vi "Prepare_Error_Array(SubVI).vi"(9 "Value":dbl, 10 "Info":dbl, 11 "Array in":string[](array[string])) -> (3 "Array out":string[](array[string]))   [LabVIEW 2017]
doc: "SubVI that update string array containing error list that i displayed on main window."
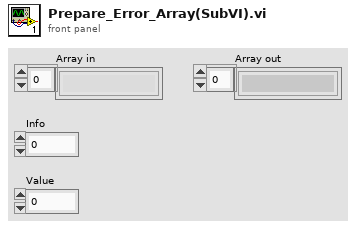
[diagram p1: front panel]
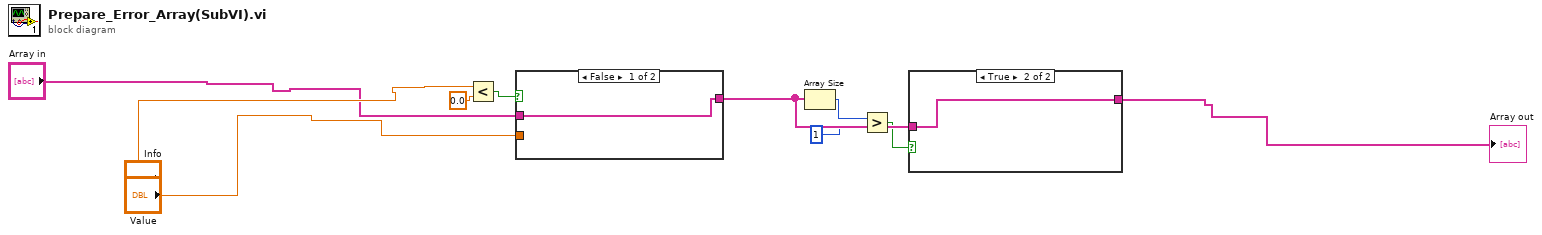
[diagram p0: block diagram]
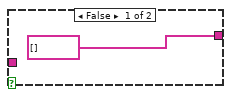
[diagram p2: hidden frame]
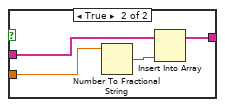
[diagram p3: hidden frame]
diagram:
  n1 = Less?(x="Info", y=0.0) -> (x < y?=w5:bool)
  n2 = case shown="False" w5 {
    tunnel: "Array in" -> [w11 w13]
    tunnel: "Value" -> [_ w15]
    tunnel: [w11 w12] -> w4
    frame False {
    }
    frame True {
      n3 = Number To Fractional String(number=w15) -> (F-format string=w14:string)  [unwired: 3 in]
      n4 = Insert Into Array(array=w13, new element=w14) -> (w12:string[])  [unwired: 1 in]
    }
  }
  n5 = Array Size(array=w4) -> (size(s)=w3:i32)
  n6 = Greater?(x=w3, y=1) -> (0:w1:bool)
  n7 = case shown="True" w1 {
    tunnel: w4 -> [_ w17]
    tunnel: [string[] [] w17] -> w10
    frame False {
    }
    frame True {
    }
  }
  "Array out" <- w10
